vi "UIRef.vi"(8 "error in":errorcluster, 11 "node in":refnum<class "TimingSource.lvclass">) -> (0 "error out":errorcluster, 2 "VI refnum":refnum<vi>, 3 "node out":refnum<class "TimingSource.lvclass">)   [LabVIEW 2015, in "TimingSource.lvclass"]
doc: "Stores the static reference to the UI of the node."
uses:
  TimingSource.lvclass
  TimingSource UI.vi
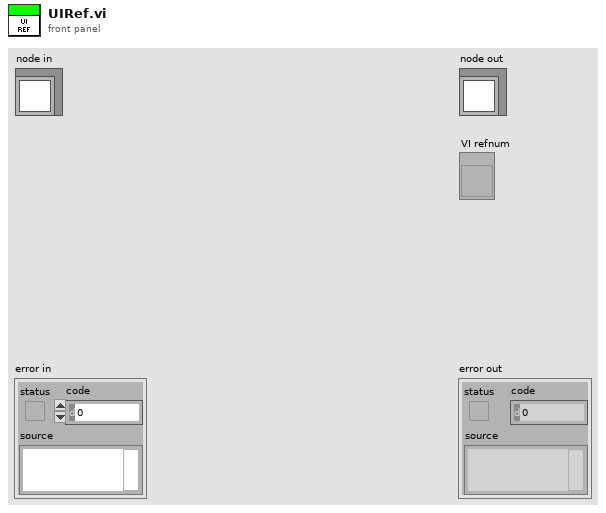
[diagram p1: front panel]
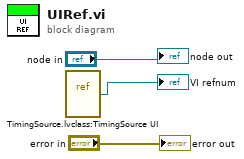
[diagram p0: block diagram]
diagram:
  n1 = vi-ref "TimingSource.lvclass:TimingSource UI.vi"() -> (→"VI refnum":refnum<vi>)
  "error out" <- "error in"
  "node out" <- "node in"
